vi "Execute.vi"(8 "error in":errorcluster, 11 "O3 Level STEP in":refnum<class "O3 Lamp Frequency STEP.lvclass">) -> (0 "error out":errorcluster, 1 "Next Step?":bool, 2 "MSG":string, 3 "O3 Level STEP out":refnum<class "O3 Lamp Frequency STEP.lvclass">)   [LabVIEW 2014, in "O3 Lamp Frequency STEP.lvclass"]
uses:
  O3 Lamp Frequency STEP.lvclass
  <vilib>/ActorFramework/Message Enqueuer/Message Enqueuer.lvclass
  Controller/Messages/Send Change Frequency MSG/Send Change Frequency MSG.lvclass
  reusable/Sequence/STEPS/LEAVES/Double/Switch DBL.lvclass/Switch DBL.ctl
  reusable/Sequence/STEPS/STEP.lvclass/STEP.ctl
  <vilib>/ActorFramework/Message Enqueuer/Message Enqueuer.lvclass/Message Enqueuer.ctl
  reusable/Sequence/STEPS/LEAVES/Double/Read val.vi
  reusable/Sequence/STEPS/Read Obj.vi
  <vilib>/ActorFramework/Message Priority Queue/Priority Enqueue.vi
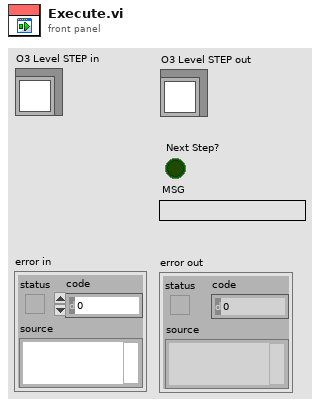
[diagram p1: front panel]
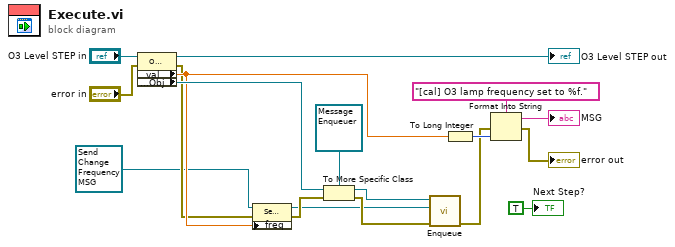
[diagram p0: block diagram]
diagram:
  n1 = property class="O3 Level"(reference="O3 Level STEP in", error in="error in") -> (reference out=→"O3 Level STEP out":refnum<class "O3 Lamp Frequency STEP.lvclass">, error out=w2:errorcluster, "val"=w6:dbl, "Accessors:Obj"=w7:refnum<class>)
  n2 = property class="Send Change Frequency MSG.lvcla"(reference=refnum<class "Send Change Frequency MSG.lvclass"> refnum ("Controller:Send Change Frequency MSG.lvclass"), error in=w2, "freq"=w6) -> (reference out=w4:refnum<class "Send Change Frequency MSG.lvclass">, error out=w5:errorcluster)
  n3 = To More Specific Class(target class=refnum<class "Message Enqueuer.lvclass"> refnum ("Message Enqueuer in"), reference=w7, error in=w5) -> (specific class reference=w8:refnum<class "Message Enqueuer.lvclass">, error out=w9:errorcluster)
  n4 = call <vilib>:"Enqueue.vi"("error in (no error)"=w9, "Message"=w4, "Message Enqueuer in"=w8) -> ("error out"=w3:errorcluster)  [unwired: 7 in, 1 out]
  n5 = To Long Integer(number=w6) -> (32bit integer=w16:i32)
  n6 = Format Into String(format string="[cal] O3 lamp frequency set to %f.", error in=w3, w16) -> (resulting string=→"MSG":string, error out=→"error out":errorcluster)  [unwired: 1 in]
  "Next Step?" <- TRUE ("Next Step?")
